vi "Generate H Matrix for Least Squares Fit.vi"(2 "[Y]":dbl[](array[numeric]), 3 "[X]":dbl[](array[numeric]), 4 "Highest order":i32) -> (0 "H":dbl[][](array[numeric]), 1 "[terms]":string[](array[string]))   [LabVIEW 2013]
doc: "This vi takes in the dependent variables X and Y and generates the matrix that represents the formula you use to fit the data set {X, Y}. H[i][j] are the function values of X[i]."
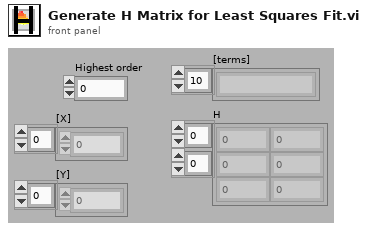
[diagram p1: front panel]
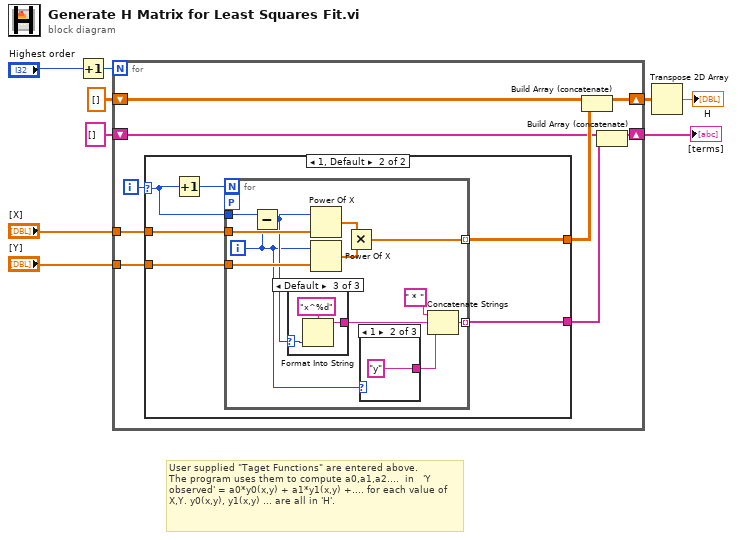
[diagram p0: block diagram]
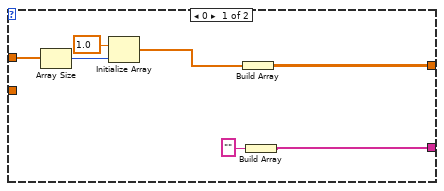
[diagram p2: hidden frame]
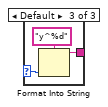
[diagram p4: hidden frame]
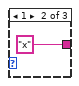
[diagram p6: hidden frame]
diagram:
  # "User supplied \"Taget Functions\" are entered above.\nThe program uses them to compute a0,a1,a2....  in   'Y observed' = a0*y0(x,y) + a1*y1(x,y) +.... for each value of X,Y. y0(x,y), y1(x,y) ... are all in 'H'."
  n1 = Increment(x="Highest order") -> (x+1=w2:i32)
  n2 = for {
    N: w2 -> [_]
    tunnel: "[X]" -> [w16]
    tunnel: "[Y]" -> [w18]
    shift-right: [w13] -> w9
    shift-left: dbl[][] [] ("transposed array") -> [w14]
    shift-right: [w11] -> w8
    shift-left: string[] [] -> [w12]
    i -> [w17]
    n3 = case shown="1, Default" w17 {
      selector: w17 -> [_ w27]
      tunnel: w18 -> [_ w31]
      tunnel: w16 -> [w24 w30]
      tunnel: [w22 w28] -> w15
      tunnel: [w19 w26] -> w10
      frame 0 {
        n4 = Array Size(array=w24) -> (size(s)=w23:i32)
        n5 = Initialize Array(1.0 ("element"), w23) -> (w21:dbl[])
        n6 = Build Array(w21) -> (w22:dbl[][])
        n7 = Build Array("" ("format string")) -> (w19:string[])
      }
      frame 1, Default {
        n8 = Increment(x=w27) -> (x+1=w29:i32)
        n9 = for {
          N: w29 -> [_]
          tunnel: w31 -> [w43]
          tunnel: w30 -> [w42]
          tunnel: w27 -> [w41]
          tunnel: [w38] -> w28 mode=indexing
          tunnel: [w37] -> w26 mode=indexing
          workers-P: _ -> [_]
          i -> [w34]
          n10 = Subtract(x=w41, y=w34) -> (x-y=w36:i32)
          n11 = case shown="Default" w36 {
            selector: w36 -> [_ _ w51]
            tunnel: [_ "x" ("format string") w49] -> w35
            frame 0 {
            }
            frame 1 {
            }
            frame Default {
              n12 = Format Into String(format string="x^%d", w51) -> (resulting string=w49:string)  [unwired: 2 in, 1 out]
            }
          }
          n13 = Power Of X(1:w42, 2:w36) -> (0:w40:dbl[])
          n14 = Power Of X(1:w43, 2:w34) -> (0:w39:dbl[])
          n15 = Multiply(x=w40, y=w39) -> (x*y=w38:dbl[])
          n16 = case shown="1" w34 {
            selector: w34 -> [_ _ w47]
            tunnel: [_ "y" ("format string") w45] -> w33
            frame 0 {
            }
            frame 1 {
            }
            frame Default {
              n17 = Format Into String(format string="y^%d", w47) -> (resulting string=w45:string)  [unwired: 2 in, 1 out]
            }
          }
          n18 = Concatenate Strings(" * " ("string"), w35, w33) -> (w37:string)
        }
      }
    }
    n19 = Build Array (concatenate)(w14, w15) -> (w13:dbl[][])
    n20 = Build Array (concatenate)(w12, w10) -> (w11:string[])
  }
  "[terms]" <- w8
  n21 = Transpose 2D Array(2D array=w9) -> (transposed array=→"H":dbl[][])
